vi "PositionForceLoop.vi"() -> ()   [LabVIEW 2013]
uses:
  <vilib>/rvi/FXPMathLib/FxpDiv/XNode/nifxpmath_Div.xnode
  <vilib>/rvi/FXPMathLib/FxpInterpret/XNode/nifxpmath_Interpret.xnode
  <vilib>/rvi/FXPMathLib/FxpDiv/simVIs/DllFxpDivTemp_sub.vi
  <vilib>/rvi/FXPMathLib/FxpDiv/subVIs/nifxpmath_Div_SimConfig.ctl
panel:
  out "y":fxp<+/-,32,1>
  out "x/y":fxp<+/-,64,32>
  in  "Actual Control Period (ticks)":u32
  in  "Sample Period (sec)":fxp<+/-,16,16>
  in  "Target Position x* (m)":fxp<+/-,16,16>
  in  "Target Force F*(N)":fxp<+/-,16,16>
  in  "Position FB x (m)":fxp<+/-,16,16>
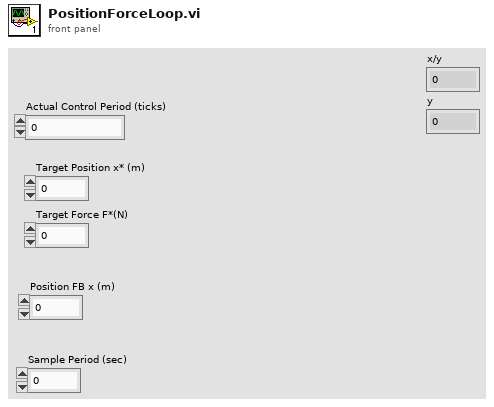
[diagram p1: front panel]
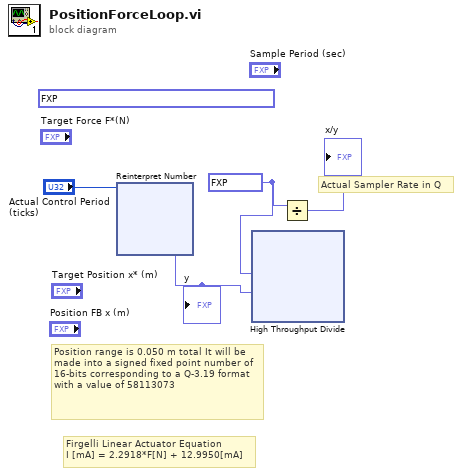
[diagram p0: block diagram]
diagram:
  (unwired) fxp<+,18,-25> 2.4999962988658808e-08
  w3 = fxp<+,17,26> 40000000.0
  # "Firgelli Linear Actuator Equation\nI [mA] = 2.2918*F[N] + 12.9950[mA]"
  # "Actual Sampler Rate in Q"
  # "Position range is 0.050 m total It will be made into a signed fixed point number of 16-bits corresponding to a Q-3.19 format with a value of 58113073"
  n1 = xnode "Reinterpret Number"("x"="Actual Control Period (ticks)") -> ("y"=w2:fxp<+/-,32,1>)
  "y" <- w2
  n2 = xnode "High Throughput Divide"("x"=w3, "y"=w2) -> ()  [unwired: 1 out]
  n3 = Divide(x=w3) -> (x/y=→"x/y":fxp<+,18,1>)  [unwired: 1 in]
